vi "LG Electrode Write To Buffer.vi"(3 "LG Electrode Grid Array":bool[][](array[boolean])=[[FALSE, FALSE, FALSE], [FALSE, FALSE, FALSE], [FALSE, FALSE, FALSE], [FALSE, FALSE, FALSE], [FALSE, FALSE, FALSE], [FALSE, FALSE, FALSE]]) -> (0 "64-bitmask Output":u64 format="%064b")   [LabVIEW 2017]
doc: "This VI will map the LG electrode grid array to ON-OFF bits in tehe 64 bit data buffer.\n\nAn array constant in this VI maps the LG electrode grid positions to the required HV channels."
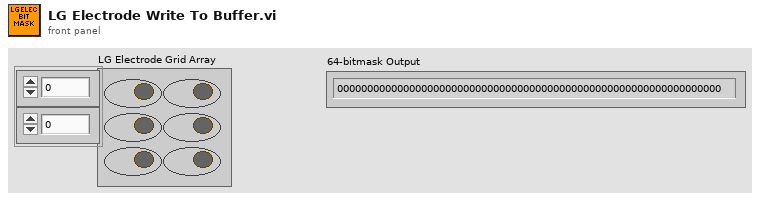
[diagram p1: front panel]
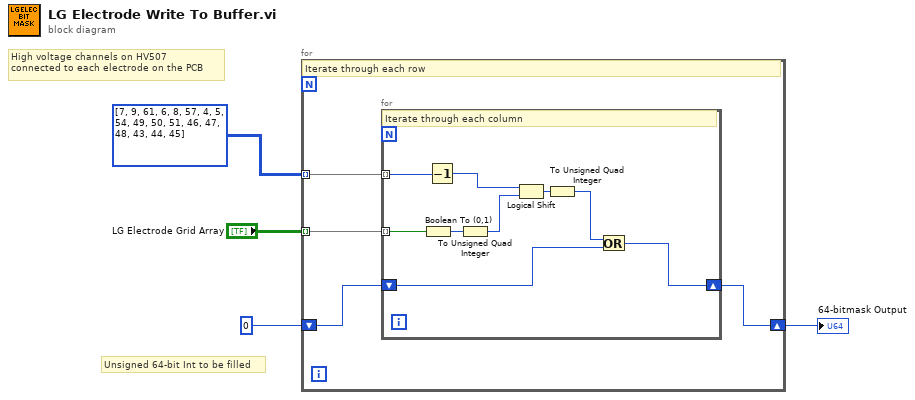
[diagram p0: block diagram]
diagram:
  # "High voltage channels on HV507\nconnected to each electrode on the PCB"
  # "Unsigned 64-bit Int to be filled"
  n1 = for {
    shift-right: [w7] -> w3
    shift-left: u64 0 -> [w8]
    tunnel: "LG Electrode Grid Array" -> [w6] mode=indexing
    tunnel: u8[][] [[7, 9, 61], [6, 8, 57], [4, 5, 54], [49, 50, 51], [46, 47, 48], [43, 44, 45]] -> [w5] mode=indexing
    # "Iterate through each row"
    n2 = for {
      shift-right: [w14] -> w7
      shift-left: w8 -> [w17]
      tunnel: w6 -> [w12] mode=indexing
      tunnel: w5 -> [w10] mode=indexing
      # "Iterate through each column"
      n3 = Boolean To (0,1)(Boolean=w12) -> (0, 1=w13:i16)
      n4 = Decrement(x=w10) -> (x-1=w9:u8)
      n5 = To Unsigned Quad Integer(1:w13) -> (0:w11:u64)
      n6 = Logical Shift(y=w9, x=w11) -> (x << y=w16:u64)
      n7 = To Unsigned Quad Integer(1:w16) -> (0:w15:u64)
      n8 = Or(x=w15, y=w17) -> (x .or. y?=w14:u64)
    }
  }
  "64-bitmask Output" <- w3
